vi "To Value.vi"(8 "error in (no error)":errorcluster, 10 "PV Data in":refnum<class "PV Data.lvclass">, 11 "NT Scalar in":refnum<class "NT Scalar.lvclass">) -> (0 "error out":errorcluster, 2 "PV Data out":refnum<class "PV Data.lvclass">, 3 "NT Scalar out":refnum<class "NT Scalar.lvclass">)   [LabVIEW 2020, in "PV Access.lvlib" / "PV Data.lvlib" / "NT Scalar.lvclass"]
uses:
  NT Scalar.lvclass
  NT Scalar.lvclass/NT Scalar.ctl
  PV Data.lvlib
  PV Data/PV Data.lvclass
  NT Base/NT Base.lvclass
  PV Data/Write Field (Variant).vi
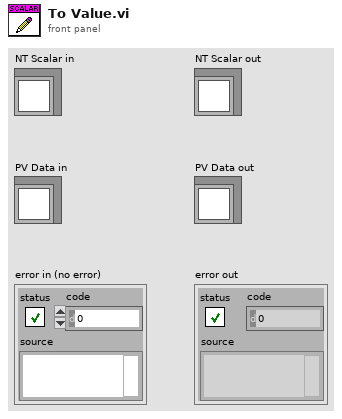
[diagram p1: front panel]
types:
  T1 = typedef "PV Access.lvlib/PV Data.lvlib/Type Code.ctl" = enum8{"Null", "Bool", "BoolA", "Int8", "Int8A", "Int16", "Int16A", "Int32", "Int32A", "Int64", "Int64A", "UInt8", "UInt8A", "UInt16", "UInt16A", "UInt32", "UInt32A", "UInt64", "UInt64A", "Float32", "Float32A", "Float64", "Float64A", "String", "StringA", "Struct", "StructA", "Union", "UnionA", "Any", "AnyA"}
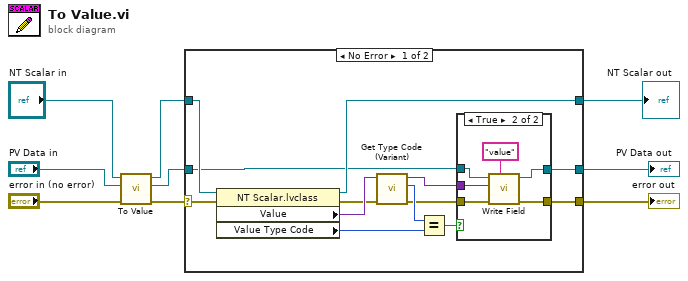
[diagram p0: block diagram]
diagram:
  n1 = call-parent "To Value.vi"("error in (no error)"="error in (no error)", "PV Data in"="PV Data in", "NT Base in"="NT Scalar in") -> ("error out"=w1:errorcluster, "PV Data out"=w2:refnum<class "PV Data.lvclass">, "NT Base out"=w3:refnum<class "NT Scalar.lvclass">)  [unwired: 6 in]
  n2 = case shown="No Error" w1 {
    selector: w1 -> [w11 w32]
    tunnel: [w15 w32] -> w9
    tunnel: [w14 w33] -> w8
    tunnel: [w13 w31] -> w7
    tunnel: w2 -> [w10 w33]
    tunnel: w3 -> [w12 w31]
    frame No Error {
      n3 = property class="NT Scalar.lvclass"(reference=w12, error in=w11) -> (reference out=w13:refnum<class "NT Scalar.lvclass">, error out=w19:errorcluster, "Value"=w22:variant, "Value Type Code"=w21:T1)
      n4 = call "Get Type Code (Variant).vi"("error in (no error)"=w19, "value"=w22) -> ("error out"=w18:errorcluster, "type code"=w20:T1, "value dup"=w17:variant)  [unwired: 5 in]
      n5 = Equal?(x=w20, y=w21) -> (x = y?=w16:bool)
      n6 = case shown="True" w16 {
        tunnel: [w24 w30] -> w15
        tunnel: [w23 w29] -> w14
        tunnel: w18 -> [w24 w27]
        tunnel: w17 -> [_ w26]
        tunnel: w10 -> [w23 w25]
        frame False {
        }
        frame True {
          n7 = call-poly "Write Field.vi"("field name"="value", "error in (no error)"=w27, "value in"=w26, "PV Data in"=w25) -> ("error out"=w30:errorcluster, "PV Data out"=w29:refnum<class "PV Data.lvclass">)  [unwired: 5 in, 1 out]
        }
      }
    }
    frame Error {
    }
  }
  "error out" <- w9
  "NT Scalar out" <- w7
  "PV Data out" <- w8
